vi "tb_10log10 SGL.vi"() -> ()   [LabVIEW 2011]
panel:
  out "Error":dbl[](graph)
  out "FXP Output":dbl[](array[numeric])
  out "LV Output":sgl[](array[numeric])
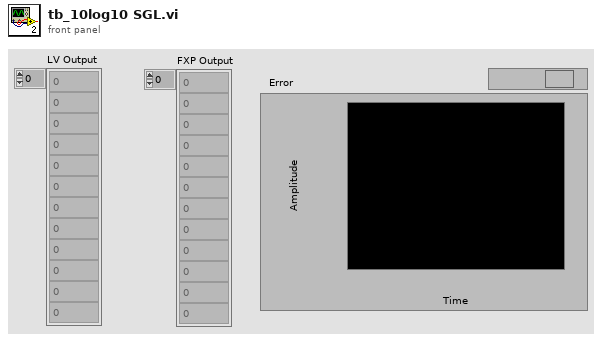
[diagram p1: front panel]
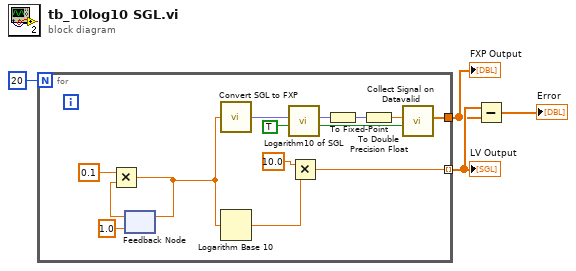
[diagram p0: block diagram]
diagram:
  n1 = for {
    N: 20 -> [_]
    tunnel: [w15] -> w3 mode=indexing
    tunnel: [w11] -> w2
    n2 = feedback #1(1.0) -> (w7:dbl)
    n3 = Multiply(x=0.1, y=w7) -> (x*y=w5:dbl)
    n4 = feedback-in #1(w5) -> ()
    n5 = call <userlib>:"Convert SGL to FXP.vi"("Input"=w5) -> ("FXP Output"=w12:fxp<+,32,32>)  [unwired: 14 in]
    n6 = Logarithm Base 10(1:w5) -> (0:w17:dbl)
    n7 = call <userlib>:"Logarithm10 of SGL.vi"("Input Valid"=TRUE, "Input Number (SGL)"=w12) -> ("Output Valid"=w9:bool, "Logarithm"=w14:fxp<+/-,34,12>)  [unwired: 6 in, 2 out]
    n8 = Multiply(x=sgl 10.0, y=w17) -> (x*y=w15:dbl)
    n9 = To Fixed-Point(number=w14) -> (fixed-point=w13:fxp<+/-,16,9>)  [unwired: 1 in]
    n10 = To Double Precision Float(number=w13) -> (double precision float=w10:dbl)
    n11 = call <userlib>:"Collect Signal on Datavalid.vi"("Data Valid"=w9, "Input"=w10) -> ("Output"=w11:dbl[])  [unwired: 9 in]
  }
  "LV Output" <- w3
  "FXP Output" <- w2
  n12 = Subtract(x=w3, y=w2) -> (x-y=→"Error":dbl[])
